vi "Configure Curve Point.vi"(0 "VISA resource name":refnum<visa-resource-name>, 5 "Curve (21)":dbl=21.0, 7 "Index (1)":dbl=1.0, 9 "Units Value (0.00000)":dbl format="%.5f", 11 "error in (no error)":errorcluster, 12 "Temperature Value (0.0000)":dbl format="%.4f") -> (4 "VISA resource name out":refnum<visa-resource-name>, 15 "error out":errorcluster)   [LabVIEW 2021, in "Lake Shore 336.lvlib"]
doc: "This VI configures a curve point. Temperature response data of a calibrated sensor must be reduced to a table of breakpoints before entering it into the instrument. Each breakpoint consist of one value in sensor units and one temperature value in Kelvin. Linear interpolation is used by the instrument to calculate temperature between breakpoints. From 2 to 200 breakpoints can be entered as a curve."
uses:
  <instrlib>/Lake Shore 336/Lake Shore 336.lvlib
  Instance           1 29Saved   Configure Curve Point .vi
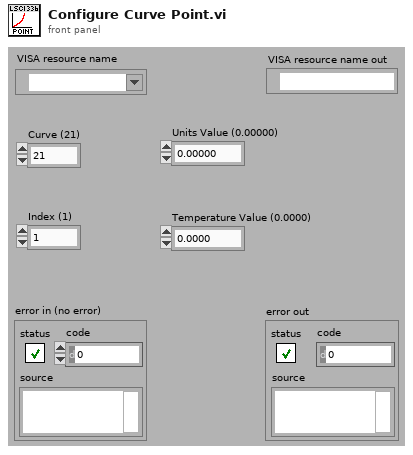
[diagram p1: front panel]
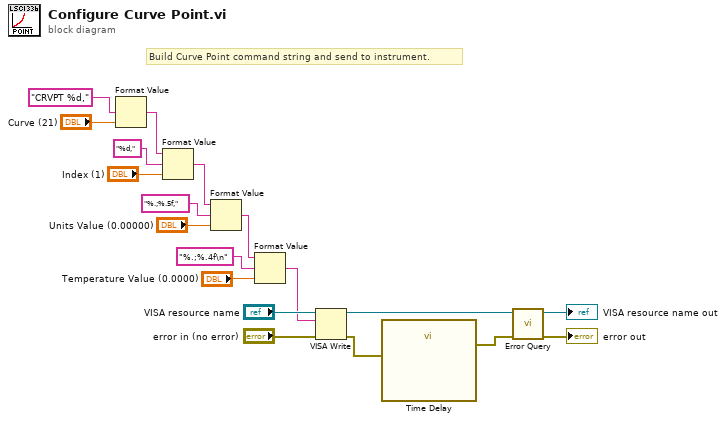
[diagram p0: block diagram]
diagram:
  # "Build Curve Point command string and send to instrument."
  n1 = Format Value(format string="CRVPT %d,", value (0)="Curve (21)") -> (output string=w8:string)  [unwired: 1 in]
  n2 = Format Value(string ("")=w8, format string="%d,", value (0)="Index (1)") -> (output string=w9:string)
  n3 = Format Value(string ("")=w9, format string="%.;%.5f,", value (0)="Units Value (0.00000)") -> (output string=w5:string)
  n4 = Format Value(string ("")=w5, format string="%.;%.4f\n", value (0)="Temperature Value (0.0000)") -> (output string=w3:string)
  n5 = VISA Write(VISA resource name="VISA resource name", write buffer=w3, error in (no error)="error in (no error)") -> (VISA resource name out=w17:refnum<visa-resource-name>, error out=w2:errorcluster)  [unwired: 1 out]
  n6 = call "Time Delay"("error in (no error)"=w2) -> ("error out"=w1:errorcluster)  [unwired: 10 in]
  n7 = call <instrlib>:"Error Query.vi"("error in (no error)"=w1, "VISA resource name"=w17) -> ("error out"=→"error out":errorcluster, "VISA resource name out"=→"VISA resource name out":refnum<visa-resource-name>)  [unwired: 7 in, 1 out]
